vi "4ByteArray2BitArray.vi"(11 "array":u8[](array[numeric])) -> (3 "Array":bool[](array[boolean]))   [LabVIEW 2012]
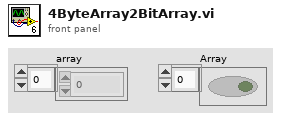
[diagram p1: front panel]
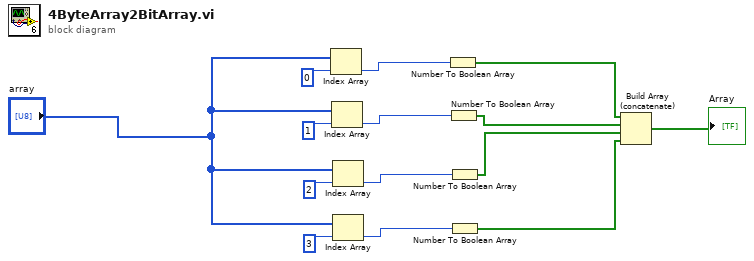
[diagram p0: block diagram]
diagram:
  n1 = Index Array(array="array", index=0) -> (element=w8:u8)
  n2 = Index Array(array="array", index=1) -> (element=w3:u8)
  n3 = Index Array(array="array", index=2) -> (element=w5:u8)
  n4 = Index Array(array="array", index=3) -> (element=w7:u8)
  n5 = Number To Boolean Array(number=w8) -> (Boolean array=w10:bool[])
  n6 = Number To Boolean Array(number=w3) -> (Boolean array=w11:bool[])
  n7 = Number To Boolean Array(number=w5) -> (Boolean array=w12:bool[])
  n8 = Number To Boolean Array(number=w7) -> (Boolean array=w13:bool[])
  n9 = Build Array (concatenate)(w10, w11, w12, w13) -> (→"Array":bool[])
